vi "合并盲元.vi"(8 "error in":errorcluster, 9 "分辨率":string, 10 "盲元数组":dbl[](array[numeric]), 11 "地址":i32=278528 format="%.0x") -> (0 "error out":errorcluster, 2 "输出盲元数组":i32[](array[numeric]))   [LabVIEW 2016]
panel:
  out "data out":u8[](array[numeric])
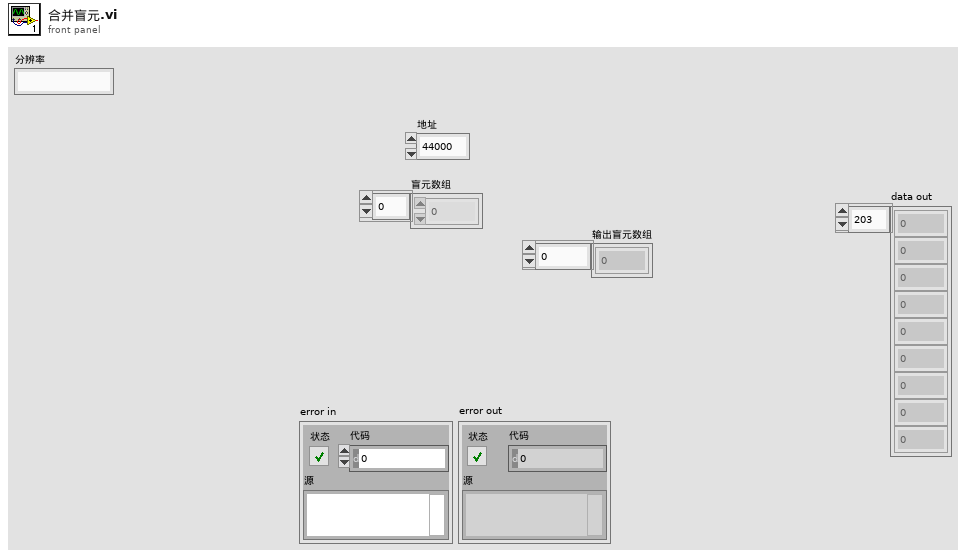
[diagram p1: front panel]
types:
  T1 = cluster{"byCmdType":u8, "bySubCmd":u8, "byPara":u8, "byAddr_h":u8, "byAddr_l":u8, "byAddr_ll":u8, "byLen_h":u8, "byLen_l":u8}
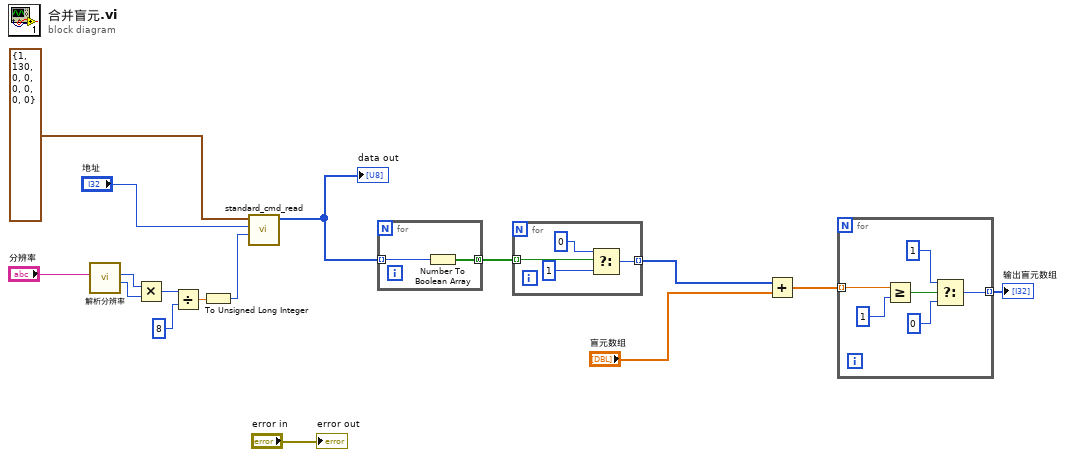
[diagram p0: block diagram]
diagram:
  n1 = call "解析分辨率.vi"("分辨率"="分辨率") -> ("number 2"=w5:i32, "number"=w6:i32)  [unwired: 9 in]
  n2 = Multiply(x=w6, y=w5) -> (x*y=w4:i32)
  n3 = Divide(x=w4, y=8) -> (x/y=w2:dbl)
  n4 = To Unsigned Long Integer(number=w2) -> (unsigned 32bit integer=w1:u32)
  n5 = call "standard_cmd_read.vi"("dwLen"=w1, "dwAddr"="地址", "cmd_std_header_t"=T1 {"byCmdType"=1, "bySubCmd"=130, "byPara"=0, "byAddr_h"=0, "byAddr_l"=0, "byAddr_ll"=0, "byLen_h"=0, "byLen_l"=0}) -> ("data out"=w13:u8[])  [unwired: 6 in, 2 out]
  "data out" <- w13
  n6 = for {
    tunnel: w13 -> [w18] mode=indexing
    tunnel: [w17] -> w12 mode=concatenating
    n7 = Number To Boolean Array(number=w18) -> (Boolean array=w17:bool[])
  }
  n8 = for {
    tunnel: w12 -> [w22] mode=indexing
    tunnel: [w19] -> w11 mode=indexing
    n9 = Select(t=0, s=w22, f=1) -> (s? t:f=w19:i32)
  }
  n10 = Add(x=w11, y="盲元数组") -> (x+y=w9:dbl[])
  n11 = for {
    tunnel: w9 -> [w28] mode=indexing
    tunnel: [w23] -> w8 mode=indexing
    n12 = Greater Or Equal?(x=w28, y=1) -> (x >= y?=w26:bool)
    n13 = Select(t=1, s=w26, f=0) -> (s? t:f=w23:i32)
  }
  "输出盲元数组" <- w8
  "error out" <- "error in"
